vi "Compute Average.vi"(8 "error in (no error)":errorcluster, 10 "Data":dbl[](array[numeric]), 11 "Video Processor in":refnum<class "Video Cam Processor.lvclass">) -> (0 "error out":errorcluster, 3 "Video Processor out":refnum<class "Video Cam Processor.lvclass">)   [LabVIEW 2018]
uses:
  Roughness Averager/Roughness Averager.lvclass
  Video Frame/Video Frame.lvclass
  Video Cam Processor.lvclass
  C:/Users/aaron.jencks/Documents/GitHub/emerson_seed_object_detection/LabVIEW/Projects/Paul's Video Viewer/Classes/Realsense Cam Video File Wrapper/Realsense Cam File Wrapper.lvclass
  C:/Users/aaron.jencks/Documents/GitHub/emerson_seed_object_detection/LabVIEW/Projects/Paul's Video Viewer/Classes/Video Processor/Video Processor.lvclass
  C:/Users/aaron.jencks/Documents/GitHub/emerson_seed_object_detection/LabVIEW/Projects/Paul's Video Viewer/Classes/Video File/Video File.lvclass
  C:/Users/aaron.jencks/Documents/GitHub/emerson_seed_object_detection/LabVIEW/Projects/Paul's Video Viewer/Classes/Standard Averager/Standard Averager.lvclass
  C:/Users/aaron.jencks/Documents/GitHub/emerson_seed_object_detection/LabVIEW/Projects/Paul's Video Viewer/Classes/Averager/Averager.lvclass
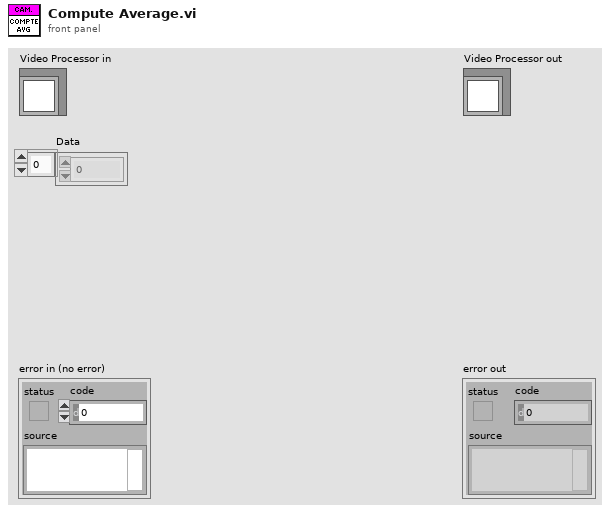
[diagram p1: front panel]
types:
  T1 = typedef "IMAQ Image.ctl" = refnum<image>
  T2 = cluster{"Normal":cluster{"Averages":cluster{"Average":dbl, "RMS":dbl, "Absolute Mean Deviation":dbl}, "Global Heuristics":cluster{"Max":dbl, "Min":dbl, "Max Peak-to-Peak":dbl}, "Skewdness":dbl, "Kurtosis":dbl, "RzDIN":dbl, "RzJIS":dbl}, "Slope Parameters":cluster{"Rdq":dbl, "Rda":dbl}, "Areal Roughness":cluster{"Peak Density":dbl}}
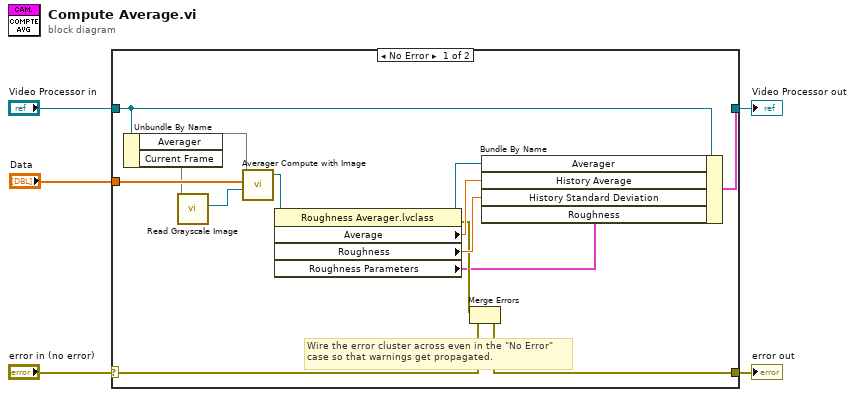
[diagram p0: block diagram]
diagram:
  n1 = case shown="No Error" "error in (no error)" {
    selector: "error in (no error)" -> [w13 w21]
    tunnel: [w12 w21] -> w4
    tunnel: [w15 w20] -> w2
    tunnel: "Video Processor in" -> [w19 w20]
    tunnel: "Data" -> [w9 _]
    frame No Error {
      # "Wire the error cluster across even in the \"No Error\"\ncase so that warnings get propagated."
      n2 = Unbundle By Name(w19) -> ("Averager"=w11, "Current Frame"=w7)
      n3 = call-dynamic "Read Grayscale Image.vi"("Video Frame in"=w7) -> ("Image"=w6:T1)  [unwired: 8 in, 2 out]
      n4 = call-dynamic "Averager Compute with Image.vi"("Grayscale Image"=w6, "Data"=w9, "Roughness Averager in"=w11) -> ("Roughness Averager out"=w10:refnum<class "Roughness Averager.lvclass">)  [unwired: 7 in, 1 out]
      n5 = property class="Roughness Averager.lvclass"(reference=w10) -> (reference out=w16:refnum<class "Roughness Averager.lvclass">, error out=w14:errorcluster, "Average"=w18:dbl, "Roughness"=w17:dbl, "Roughness Parameters"=w8:T2)  [unwired: 1 in]
      n6 = Merge Errors(w14, w13) -> (w12:errorcluster)
      n7 = Bundle By Name(cluster=w19, "Averager"=w16, "History Average"=w18, "History Standard Deviation"=w17, "Roughness"=w8) -> (w15:cluster{})
    }
    frame Error {
    }
  }
  "error out" <- w4
  "Video Processor out" <- w2
